vi "Команда обмена 255 (Команда запроса на обновление данных) (SubVI).vi"(7 "error in":errorcluster) -> (23 "Кластер параметров 255-ой команды":T1, 27 "error out":errorcluster)   [LabVIEW 2013]
doc: "255 команда - команда на обновление данных по мишеням"
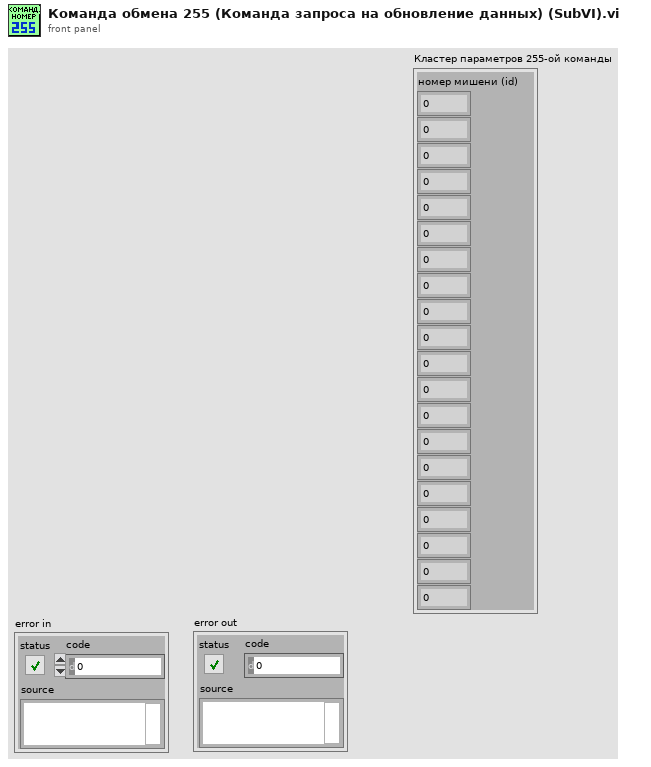
[diagram p1: front panel]
types:
  T1 = cluster{"номер мишени (id)":u8, u8, u8, u8, u8, u8, u8, u8, u8, u8, u8, u8, u8, u8, u8, u8, u8, u8, u8, u8}
  T2 = cluster{"Команда на обновление данных по всем мишеням":u8, u8, u8, u8, u8, u8, u8, u8, u8, u8, u8, u8, u8, u8, u8, u8, u8, u8, u8, u8}
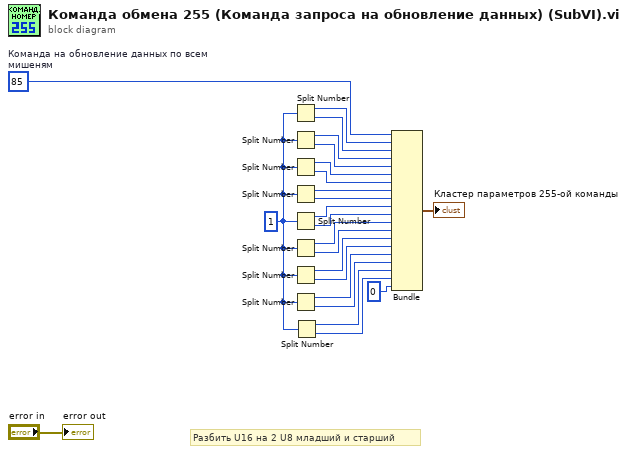
[diagram p0: block diagram]
diagram:
  w2 = u8 1
  w6 = u8 85  # Команда на обновление данных по всем мишеням
  # "Разбить U16 на 2 U8 младший и старший"
  n1 = Split Number(x=w2) -> (hi(x)=w5:u8, lo(x)=w4:u8)
  n2 = Split Number(x=w2) -> (hi(x)=w7:u8, lo(x)=w8:u8)
  n3 = Split Number(x=w2) -> (hi(x)=w9:u8, lo(x)=w10:u8)
  n4 = Split Number(x=w2) -> (hi(x)=w11:u8, lo(x)=w12:u8)
  n5 = Split Number(x=w2) -> (hi(x)=w13:u8, lo(x)=w14:u8)
  n6 = Split Number(x=w2) -> (hi(x)=w15:u8, lo(x)=w16:u8)
  n7 = Split Number(x=w2) -> (hi(x)=w17:u8, lo(x)=w18:u8)
  n8 = Split Number(x=w2) -> (hi(x)=w19:u8, lo(x)=w20:u8)
  n9 = Split Number(x=w2) -> (hi(x)=w21:u8, lo(x)=w22:u8)
  n10 = Bundle("Команда на обновление данных по всем мишеням"=w6, w5, w4, w7, w8, w9, w10, w11, w12, w13, w14, w15, w16, w17, w18, w19, w20, w21, w22, u8 0) -> (→"Кластер параметров 255-ой команды":T2)  [unwired: 1 in]
  "error out" <- "error in"
